vi "initialize.vi"(0 "HGF_VISADevice":refnum<class "HGF_VISADevice.lvclass">, 3 "initializationData":variant, 5 "error in (no error)":errorcluster, 7 "binaryString":string, 8 "I8 Array":i8[](array[numeric]), 9 "prependSize? (T)":bool, 11 "byteOrder (0:big-endian, network order)":T1(ring)) -> (14 "dup HGF_VISADevice":refnum<class "HGF_VISADevice.lvclass">, 17 "found?":bool, 19 "error out":errorcluster)   [LabVIEW 2014, in "HGF_DeviceBaseClasses.lvlib" / "HGF_VISADevice.lvclass"]
doc: "This is a dynamic dispatch VI to be implemented by child classes to initialize their attributes.\n\n<B>Recommendation:</B> Use Variant for initialization data."
uses:
  HGF_VISADevice.lvclass
  HGF_DeviceBase/HGF_DeviceBase.lvclass
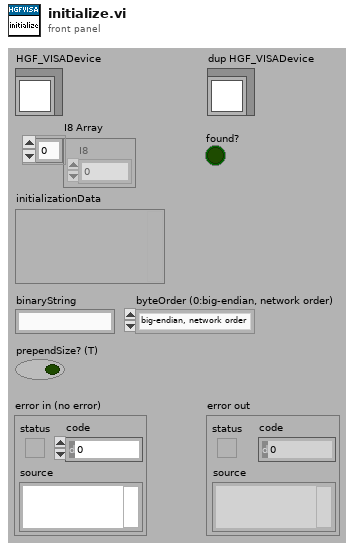
[diagram p1: front panel]
types:
  T1 = enum16{"big-endian, network order", "native, host order", "little-endian"}
  T2 = cluster{"Baud Rate":u32, "Flow Control":u16, "Parity":u16, "Data Bits":u16, "Stop Bits":u16}
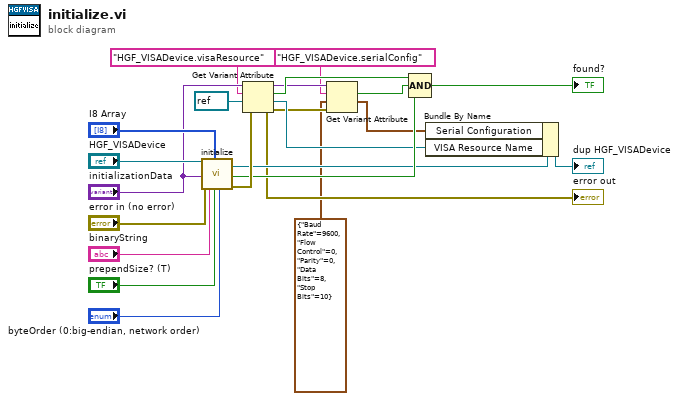
[diagram p0: block diagram]
diagram:
  n1 = call-parent "initialize.vi"("HGF_DeviceBase"="HGF_VISADevice", "initializationData"="initializationData", "error in (no error)"="error in (no error)", "binaryString"="binaryString", "I8 Array"="I8 Array", "prependSize? (T)"="prependSize? (T)", "byteOrder (0:big-endian, network order)"="byteOrder (0:big-endian, network order)") -> ("dup HGF_DeviceBase"=w9:refnum<class "HGF_VISADevice.lvclass">, "found?"=w12:bool, "error out"=w15:errorcluster)  [unwired: 10 out]
  n2 = Get Variant Attribute(Variant="initializationData", name="HGF_VISADevice.visaResource", default value (empty Variant)=refnum<visa-resource-name> refnum ("VISA Resource Name"), error in=w15) -> (duplicate Variant=w6:variant, found=w13:bool, value=w10:refnum<visa-resource-name>, error out=w5:errorcluster)
  "error out" <- w5
  n3 = Get Variant Attribute(Variant=w6, name="HGF_VISADevice.serialConfig", default value (empty Variant)=T2 {"Baud Rate"=9600, "Flow Control"=0, "Parity"=0, "Data Bits"=8, "Stop Bits"=10} ("Serial Configuration"), error in=w5) -> (found=w2:bool, value=w1:T2)  [unwired: 2 out]
  n4 = Compound Arithmetic op=AND(w13, w2, w12) -> (→"found?":bool)
  n5 = Bundle By Name(cluster=w9, "Serial Configuration"=w1, "VISA Resource Name"=w10) -> (→"dup HGF_VISADevice":refnum<class "HGF_VISADevice.lvclass">)
